vi "remove.volume.from.folder.map.vi"(10 "sortable name":string, 11 "folder map in":map{i32, map{string, i32}}(c390)) -> (3 "folder map out":map{i32, map{string, i32}}(c390))   [LabVIEW 2024, in "manager_daemon.lvclass"]
uses:
  manager_daemon.lvclass
  manager_daemon.lvclass/manager_daemon.ctl
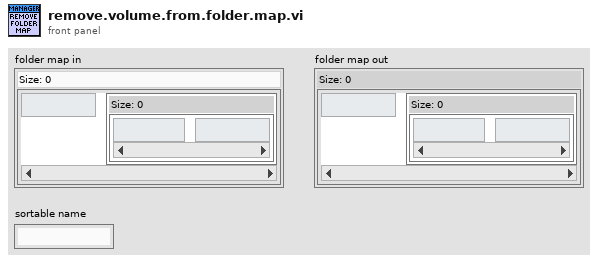
[diagram p1: front panel]
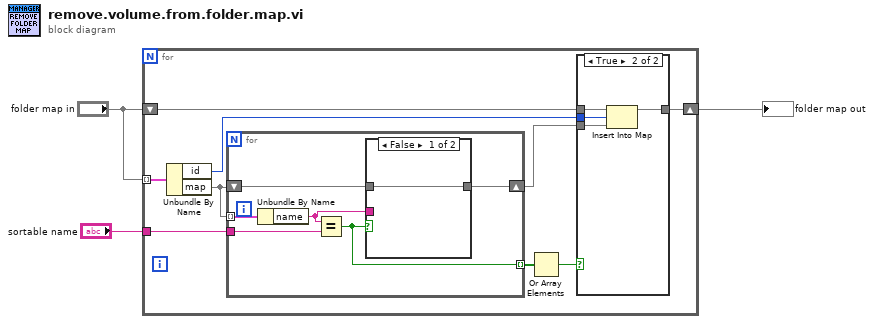
[diagram p0: block diagram]
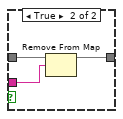
[diagram p3: hidden frame]
diagram:
  n1 = for {
    shift-right: [w6] -> w1
    shift-left: "folder map in" -> [w7]
    tunnel: "folder map in" -> [w12] mode=indexing
    tunnel: "sortable name" -> [w10]
    n2 = Unbundle By Name(w12) -> ("id"=w4:i32, "map"=w11:map{string, i32})
    n3 = for {
      shift-right: [w19] -> w5
      shift-left: w11 -> [w21]
      tunnel: w11 -> [w23] mode=indexing
      tunnel: w10 -> [w22]
      tunnel: [w18] -> w9 mode=indexing
      n4 = Unbundle By Name(w23) -> ("name"=w20:string)
      n5 = Equal?(x=w20, y=w22) -> (x = y?=w18:bool)
      n6 = case shown="False" w18 {
        tunnel: w21 -> [w24 w27]
        tunnel: w20 -> [_ w26]
        tunnel: [w24 w25] -> w19
        frame False {
        }
        frame True {
          n7 = Remove From Map(10:w26, 11:w27) -> (3:w25:map{string, i32})  [unwired: 2 out]
        }
      }
    }
    n8 = Or Array Elements(Boolean array=w9) -> (logical OR=w8:bool)
    n9 = case shown="True" w8 {
      tunnel: w7 -> [w13 w17]
      tunnel: [w13 w16] -> w6
      tunnel: w5 -> [_ w15]
      tunnel: w4 -> [_ w14]
      frame False {
      }
      frame True {
        n10 = Insert Into Map(map in=w17, key=w14, value=w15) -> (map out=w16:map{i32, map{string, i32}})  [unwired: 2 out]
      }
    }
  }
  "folder map out" <- w1
